vi "mono_imu.vi"(5 "Sensor Connections":T2(array[cluster])) -> (0 "error out":errorcluster, 1 "imu_sample":T1, 2 "tcp_out":refnum<k5>)   [LabVIEW 2018]
panel:
  in  "checksum":sgl
  in  "timer":dbl format="%#_13g"
  in  "angle_rate_z":dbl format="%#_13g"
  in  "angle_rate_y":dbl format="%#_13g"
  in  "angle_rate_x":u8
  in  "accel_z":u16
  in  "accel_y":u16
  in  "accel_x":u8
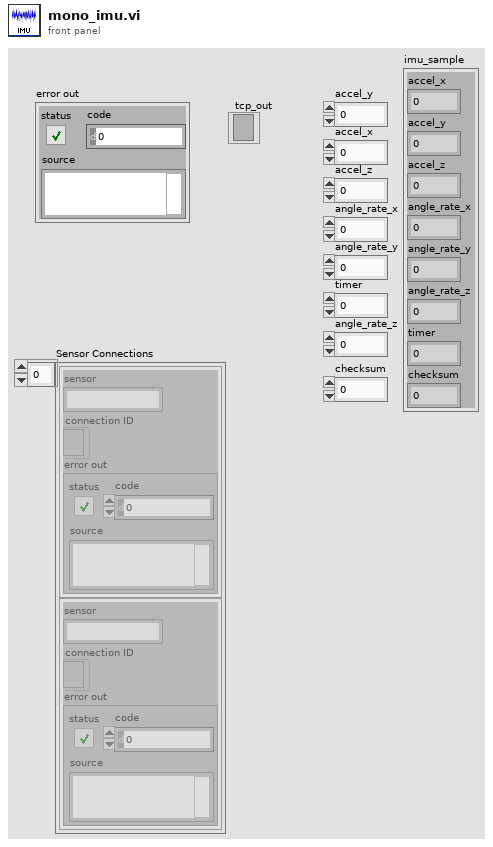
[diagram p1: front panel]
types:
  T1 = cluster{"accel_x":u8, "accel_y":u16, "accel_z":u16, "angle_rate_x":u8, "angle_rate_y":dbl, "angle_rate_z":dbl, "timer":dbl, "checksum":sgl}
  T2 = cluster{"sensor":string, "connection ID":refnum<k5>, "error out":errorcluster}[]
  T3 = cluster{"sensor":string, "connection ID":refnum<k5>, "error out":errorcluster}
  T4 = cluster{cluster{"length":u32, "time_stamp":u32, "game_time":sgl}, "data out":string}
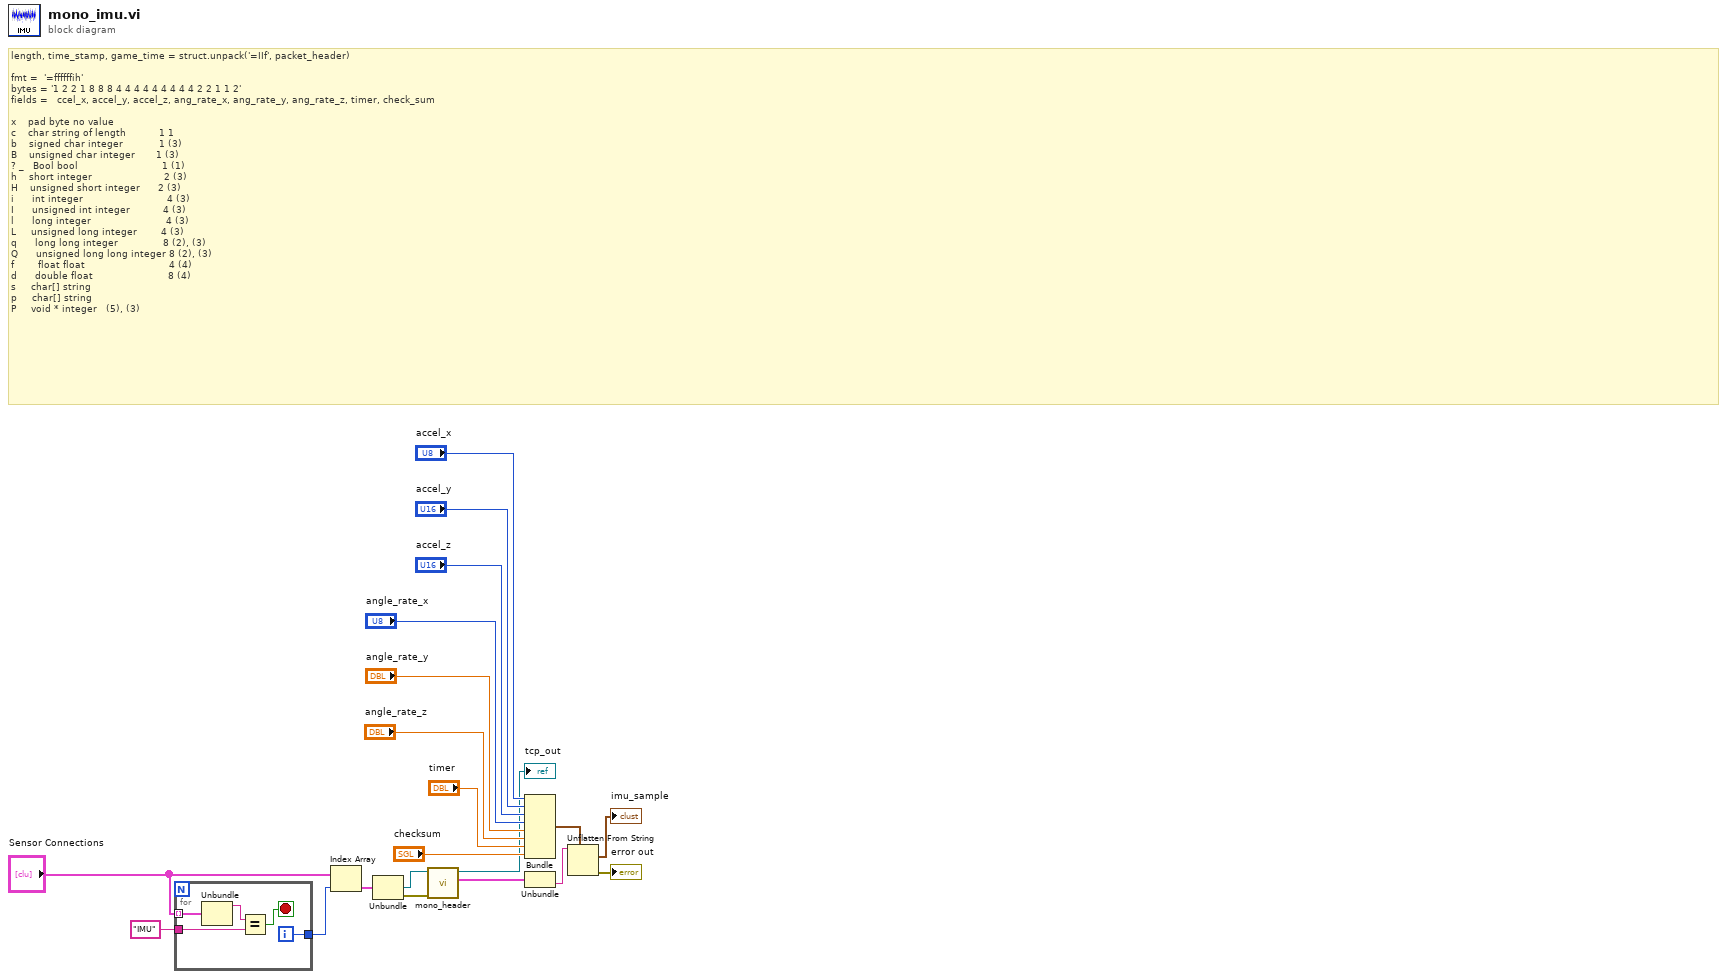
[diagram p0: block diagram]
diagram:
  # "length, time_stamp, game_time = struct.unpack('=IIf', packet_header)\n\nfmt =  '=ffffffih'\nbytes = '1 2 2 1 8 8 8 4 4 4 4 4 4 4 4 4 2 2 1 1 2'\nfields =   ccel_x, accel_y, accel_z, ang_rate_x, ang_rate_y, ang_rate_z, timer, check_sum\n\nx\t   pad byte\tno value\t \t \nc\t   char\tstring of length           1\t1\t \nb\t   signed char\tinteger\t           1\t(3)\nB\t   unsigned char\tinteger\t      1\t(3)\n?\t_   Bool\tbool\t                           1\t(1)\nh\t   short\tinteger\t                       2\t(3)\nH\t   unsigned short\tinteger\t     2\t(3)\ni\t     int\tinteger\t                           4\t(3)\nI\t     unsigned int\tinteger\t          4\t(3)\nl     \tlong\tinteger\t                        4\t(3)\nL\t    unsigned long\tinteger\t       4\t(3)\nq     \tlong long\tinteger\t              8\t(2), (3)\nQ\t     unsigned long long\tinteger\t8\t(2), (3)\nf       \tfloat\tfloat\t                           4\t(4)\nd     \tdouble\tfloat\t                        8\t(4)\ns\t    char[]\tstring\t \t \np\t    char[]\tstring\t \t \nP\t    void *\tinteger\t \t(5), (3)"
  n1 = for {
    tunnel: "Sensor Connections" -> [w25] mode=indexing
    tunnel: "IMU" -> [w23]
    tunnel: [w21] -> w6
    i -> [w21]
    stop <- w22 stop-if-true
    n2 = Unbundle(w25) -> ("sensor"=w24:string)  [unwired: 2 out]
    n3 = Equal?(x=w24, y=w23) -> (x = y?=w22:bool)
  }
  n4 = Index Array(array="Sensor Connections", index=w6) -> (element=w10:T3)
  n5 = Unbundle(w10) -> ("connection ID"=w8:refnum<k5>, "error out"=w7:errorcluster)  [unwired: 1 out]
  n6 = call "mono_header.vi"("error in"=w7, "connection ID"=w8) -> ("sensor_sample"=w11:T4, "connection ID out"=→"tcp_out":refnum<k5>)  [unwired: 7 in, 1 out]
  n7 = Bundle("accel_x"="accel_x", "accel_y"="accel_y", "accel_z"="accel_z", "angle_rate_x"="angle_rate_x", "angle_rate_y"="angle_rate_y", "angle_rate_z"="angle_rate_z", "timer"="timer", "checksum"="checksum") -> (w20:T1)  [unwired: 1 in]
  n8 = Unbundle(w11) -> ("data out"=w2:string)  [unwired: 1 out]
  n9 = Unflatten From String(type=w20, binary string=w2) -> (value=→"imu_sample":T1, error out=→"error out":errorcluster)  [unwired: 3 in, 1 out]
